vi "485 comm Initialization VI.vi"(8 "error in (no error)":errorcluster, 10 "Custom XML":string, 11 "Device Item Ref in":T1 format="%.0x") -> (0 "error out":errorcluster, 3 "Device Item Ref out":T1 format="%.0x")   [LabVIEW 2015, in "485 comm Custom Device.lvlib"]
uses:
  485 comm Custom Device.lvlib
  <vilib>/NI Veristand/Custom Device API/Custom Device API.lvlib
  <vilib>/NI Veristand/Custom Device API/Custom Device Channel Type.ctl
  <vilib>/NI Veristand/Custom Device API/Custom Device Channel.ctl
  Serial - Settings.ctl
  <vilib>/NI Veristand/Custom Device API/Set Item Property (U32).vi
  <vilib>/NI Veristand/Custom Device API/Set Item Property (Variant).vi
  <vilib>/NI Veristand/Custom Device API/Set Item Property (String).vi
  <vilib>/NI Veristand/Custom Device API/Set Item Property (U16).vi
  <vilib>/NI Veristand/Custom Device API/Set Item Property (Boolean).vi
  <vilib>/NI Veristand/Custom Device API/Custom Device Item Ref.ctl
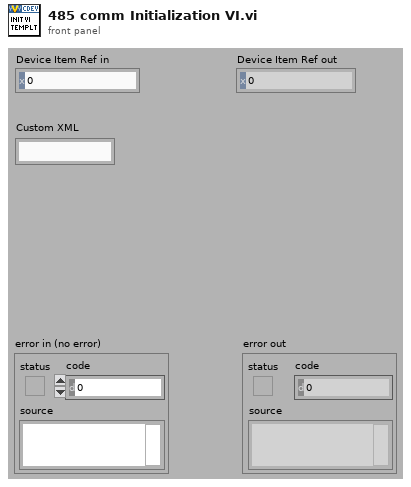
[diagram p1: front panel]
types:
  T1 = typedef "Custom Device API.lvlib/Custom Device Item Ref.ctl" = u64
  T2 = typedef "485 comm Custom Device.lvlib/Serial - Settings.ctl" = cluster{"baud rate":u32, "data bits":u16, "parity":enum16{"None", "Odd", "Even", "Mark", "Space"}, "stop bits":u16, "flow control":u16}
  T3 = typedef "Custom Device API.lvlib/Custom Device Channel.ctl" = cluster{"Type":T4, "Units":string, "Default Value":dbl, "Faultable":bool, "Scalable":bool}
  T4 = typedef "Custom Device API.lvlib/Custom Device Channel Type.ctl" = enum16{"Input", "Output"}
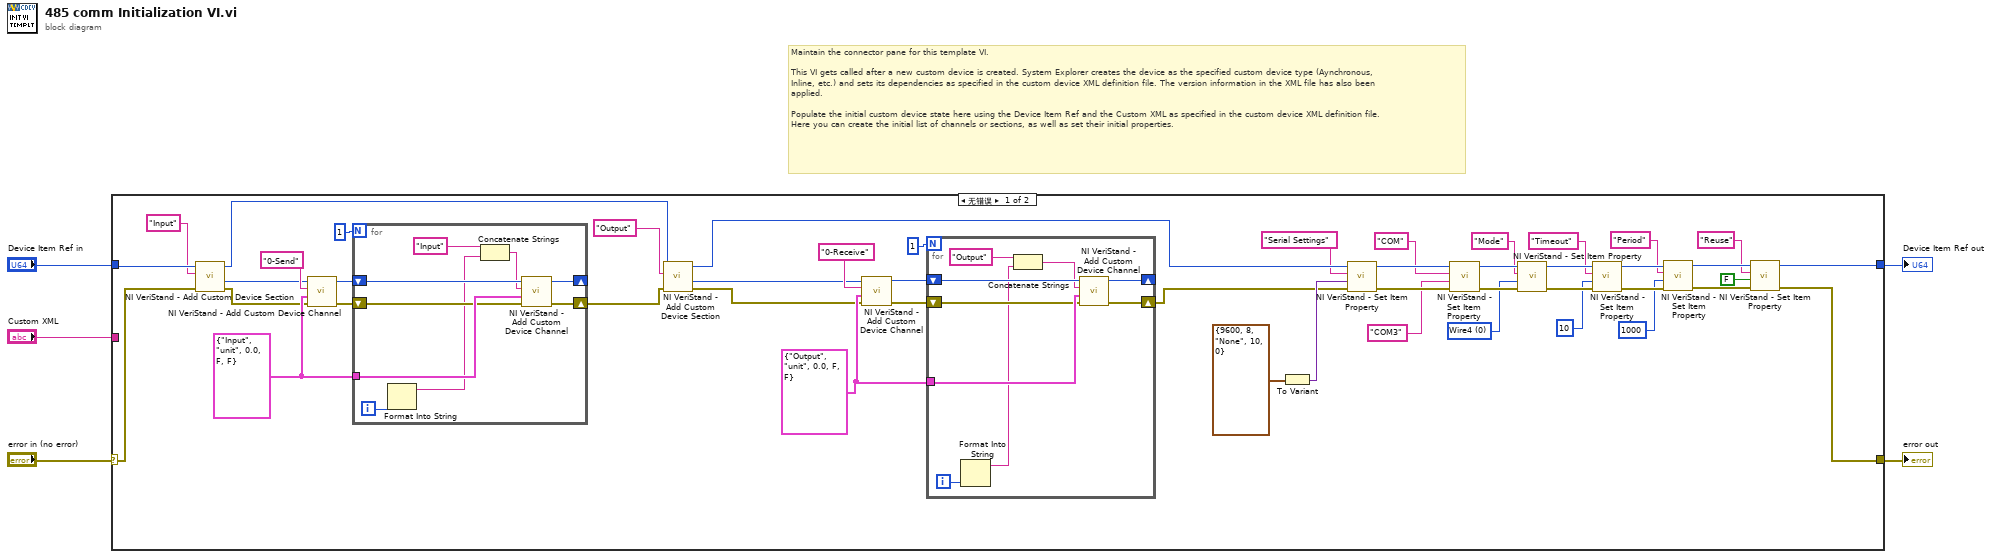
[diagram p0: block diagram]
diagram:
  # "Maintain the connector pane for this template VI.\n\nThis VI gets called after a new custom device is created. System Explorer creates the device as the specified custom device type (Aynchronous, Inline, etc.) and sets its dependencies as specified in the custom device XML definition file. The version information in the XML file has also been applied.\n\nPopulate the initial custom device state here using the Device Item Ref and the Custom XML as specified in the custom device XML definition file. Here you can create the initial list of channels or sections, as well as set their initial properties."
  n1 = case shown="无错误" "error in (no error)" {
    selector: "error in (no error)" -> [w45 w72]
    tunnel: [w25 w72] -> w5
    tunnel: [w27 w71] -> w3
    tunnel: "Device Item Ref in" -> [w52 w71]
    tunnel: "Custom XML" -> [_ _]
    frame No Error {
      w37 = u16 0 items=["Wire4", "Wire2-EchoDTR", "Wire2-CtrlDTR", "Wire2-Auto"] ("RS-485 Transceiver Mode 2")
      w16 = T3 {"Type"=enum."Output", "Units"="unit", "Default Value"=0.0, "Faultable"=FALSE, "Scalable"=FALSE} ("Channel")
      w20 = T3 {"Type"=enum."Input", "Units"="unit", "Default Value"=0.0, "Faultable"=FALSE, "Scalable"=FALSE} ("Channel")
      n2 = call <vilib>:"NI VeriStand - Add Custom Device Section.vi"("error in (no error)"=w45, "Section Name"="Input", "Parent Ref in"=w52) -> ("error out"=w15:errorcluster, "Section Ptr"=w13:T1, "Parent Ref out"=w21:T1)  [unwired: 5 in, 1 out]
      n3 = call <vilib>:"NI VeriStand - Add Custom Device Channel.vi"("error in (no error)"=w15, "Channel"=w20, "Channel Name"="0-Send", "Parent Ref in"=w13) -> ("error out"=w14:errorcluster, "Parent Ref out"=w12:T1)  [unwired: 4 in, 2 out]
      n4 = for {
        N: 1 -> [_]
        tunnel: w20 -> [w70]
        shift-right: [w63] -> _
        shift-left: w12 -> [w69]
        shift-right: [w62] -> w11
        shift-left: w14 -> [w68]
        i -> [w66]
        n5 = Format Into String(w66) -> (resulting string=w65:string)  [unwired: 3 in, 1 out]
        n6 = Concatenate Strings("Input" ("Channel Name"), w65) -> (w64:string)
        n7 = call <vilib>:"NI VeriStand - Add Custom Device Channel.vi"("error in (no error)"=w68, "Channel"=w70, "Channel Name"=w64, "Parent Ref in"=w69) -> ("error out"=w62:errorcluster, "Parent Ref out"=w63:T1)  [unwired: 4 in, 2 out]
      }
      n8 = call <vilib>:"NI VeriStand - Add Custom Device Section.vi"("error in (no error)"=w11, "Section Name"="Output", "Parent Ref in"=w21) -> ("error out"=w9:errorcluster, "Section Ptr"=w7:T1, "Parent Ref out"=w50:T1)  [unwired: 5 in, 1 out]
      n9 = call <vilib>:"NI VeriStand - Add Custom Device Channel.vi"("error in (no error)"=w9, "Channel"=w16, "Channel Name"="0-Receive", "Parent Ref in"=w7) -> ("error out"=w8:errorcluster, "Parent Ref out"=w6:T1)  [unwired: 4 in, 2 out]
      n10 = for {
        N: 1 -> [_]
        tunnel: w16 -> [w61]
        shift-right: [w60] -> _
        shift-left: w6 -> [w59]
        shift-right: [w58] -> w10
        shift-left: w8 -> [w57]
        i -> [w56]
        n11 = Format Into String(w56) -> (resulting string=w55:string)  [unwired: 3 in, 1 out]
        n12 = Concatenate Strings("Output" ("Channel Name"), w55) -> (w53:string)
        n13 = call <vilib>:"NI VeriStand - Add Custom Device Channel.vi"("error in (no error)"=w57, "Channel"=w61, "Channel Name"=w53, "Parent Ref in"=w59) -> ("error out"=w58:errorcluster, "Parent Ref out"=w60:T1)  [unwired: 4 in, 2 out]
      }
      n14 = To Variant(anything=T2 {"baud rate"=9600, "data bits"=8, "parity"=enum."None", "stop bits"=10, "flow control"=0} ("Serial Settings")) -> (Variant=w46:variant)
      n15 = call-poly <vilib>:"NI VeriStand - Set Item Property.vi"("error in (no error)"=w10, "Value"=w46, "Property Name"="Serial Settings", "Item Ref in"=w50) -> ("error out"=w42:errorcluster, "Item Ref out"=w44:T1)  [unwired: 5 in, 1 out]
      n16 = call-poly <vilib>:"NI VeriStand - Set Item Property.vi"("error in (no error)"=w42, "Value"="COM3", "Property Name"="COM", "Item Ref in"=w44) -> ("error out"=w39:errorcluster, "Item Ref out"=w40:T1)  [unwired: 5 in, 1 out]
      n17 = call-poly <vilib>:"NI VeriStand - Set Item Property.vi"("error in (no error)"=w39, "Value"=w37, "Property Name"="Mode", "Item Ref in"=w40) -> ("error out"=w35:errorcluster, "Item Ref out"=w36:T1)  [unwired: 5 in, 1 out]
      n18 = call-poly <vilib>:"NI VeriStand - Set Item Property.vi"("error in (no error)"=w35, "Value"=u32 10, "Property Name"="Timeout", "Item Ref in"=w36) -> ("error out"=w31:errorcluster, "Item Ref out"=w32:T1)  [unwired: 5 in, 1 out]
      n19 = call-poly <vilib>:"NI VeriStand - Set Item Property.vi"("error in (no error)"=w31, "Value"=u32 1000, "Property Name"="Period", "Item Ref in"=w32) -> ("error out"=w26:errorcluster, "Item Ref out"=w28:T1)  [unwired: 5 in, 1 out]
      n20 = call-poly <vilib>:"NI VeriStand - Set Item Property.vi"("error in (no error)"=w26, "Value"=FALSE, "Property Name"="Reuse", "Item Ref in"=w28) -> ("error out"=w25:errorcluster, "Item Ref out"=w27:T1)  [unwired: 5 in, 1 out]
    }
    frame Error {
    }
  }
  "error out" <- w5
  "Device Item Ref out" <- w3
